vi "Update WheelAngle.vi"(2 "error in (no error)":errorcluster, 3 "Time Since Last Update":dbl, 4 "Car.lvclass":refnum<class "Car.lvclass">) -> (0 "error out":errorcluster, 1 "Car.lvclass 2":refnum<class "Car.lvclass">)   [LabVIEW 2015, in "Car.lvclass"]
uses:
  Car.lvclass
  Car.lvclass/Car.ctl
panel:
  in  "Wheel Angle Change Rate":dbl=10.0
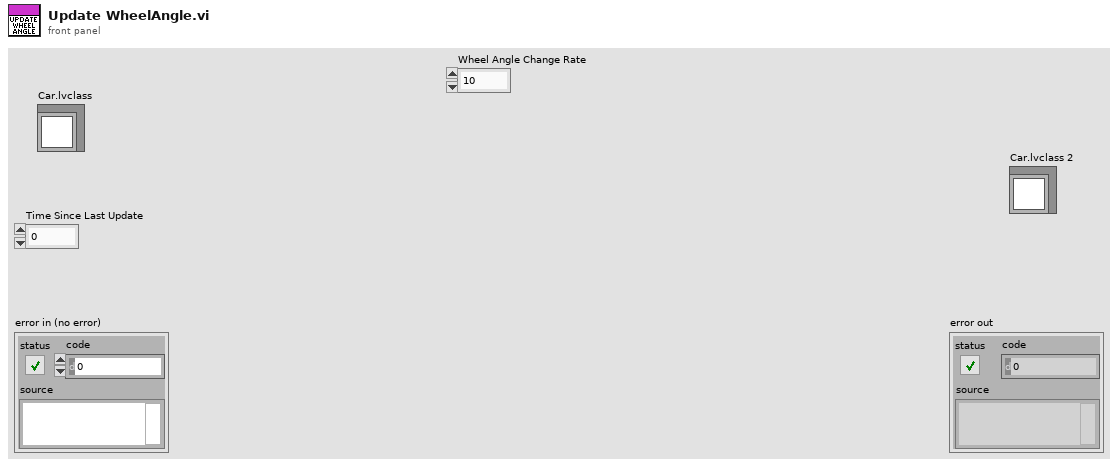
[diagram p1: front panel]
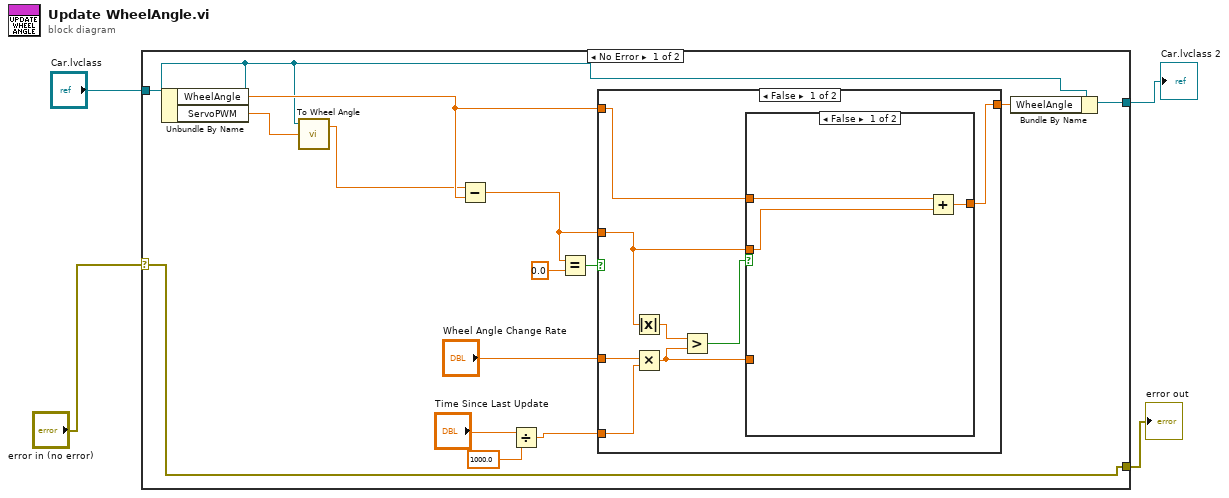
[diagram p0: block diagram]
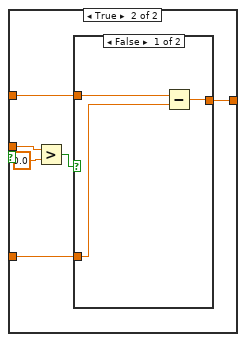
[diagram p2: hidden frame]
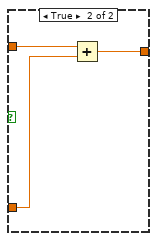
[diagram p3: hidden frame]
diagram:
  n1 = case shown="No Error" "error in (no error)" {
    selector: "error in (no error)" -> [w18 w44]
    tunnel: [w18 w44] -> w3
    tunnel: [w17 w43] -> w2
    tunnel: "Car.lvclass" -> [w6 w43]
    frame No Error {
      n2 = Unbundle By Name(w6) -> ("WheelAngle"=w13:dbl, "ServoPWM"=w7:dbl)
      n3 = call "To Wheel Angle.vi"("Servo PWM"=w7, "Car.lvclass"=w6) -> ("Wheel Angle"=w5:dbl)  [unwired: 1 in, 1 out]
      n4 = Subtract(x=w5, y=w13) -> (x-y=w11:dbl)
      n5 = Divide(x="Time Since Last Update", y=1000.0) -> (x/y=w9:dbl)
      n6 = Equal?(x=w11, y=0.0) -> (x = y?=w16:bool)
      n7 = case shown="False" w16 {
        tunnel: [w19 w42] -> w14
        tunnel: w13 -> [w21 w42]
        tunnel: "Wheel Angle Change Rate" -> [w26 _]
        tunnel: w9 -> [w25 _]
        tunnel: w11 -> [w22 _]
        frame False {
          n8 = Absolute Value(x=w22) -> (abs(x)=w24:dbl)
          n9 = Multiply(x=w26, y=w25) -> (x*y=w20:dbl)
          n10 = Greater?(x=w24, y=w20) -> (0:w23:bool)
          n11 = case shown="False" w23 {
            tunnel: w22 -> [w27 w35]
            tunnel: w21 -> [w28 w32]
            tunnel: w20 -> [_ w31]
            tunnel: [w29 w30] -> w19
            frame False {
              n12 = Add(x=w28, y=w27) -> (x+y=w29:dbl)
            }
            frame True {
              n13 = Greater?(x=w35, y=0.0) -> (0:w33:bool)
              n14 = case shown="False" w33 {
                tunnel: w32 -> [w37 w41]
                tunnel: w31 -> [w36 w40]
                tunnel: [w38 w39] -> w30
                frame False {
                  n15 = Subtract(x=w37, y=w36) -> (x-y=w38:dbl)
                }
                frame True {
                  n16 = Add(x=w41, y=w40) -> (x+y=w39:dbl)
                }
              }
            }
          }
        }
        frame True {
        }
      }
      n17 = Bundle By Name(cluster=w6, "WheelAngle"=w14) -> (w17:refnum<class "Car.lvclass">)
    }
    frame Error {
    }
  }
  "Car.lvclass 2" <- w2
  "error out" <- w3
